vi "PicoScope6000ExampleBlockAdvancedTrigger.vi"() -> ()   [LabVIEW 2010]
uses:
  shared/PicoBuffers.ctl
  shared/Buffer and Transfer Settings.ctl
  shared/Acquisition Settings.ctl
  PicoScope6000Lib/PicoScope6000AnalogChannelSettings.ctl
panel:
  in  "Pulse Width Qualifier Settings":T1={"Direction"=2, "Lower Limit"=0, "Upper Limit"=0, "Pulse Width Type"=4} {"Pulse Width Type" items=["None", "Less Than", "Greater Than", "In Range", "Out of Range"]; "Direction" items=["Rising"=2, "Falling"=3, "Rising Lower"=7, "Falling Lower"=8]}
  in  "Pulse Width Qualifier Conditions":T2 {"Condition Logic" items=["AND", "OR", "XOR"]}
  in  "Trigger Conditions":T3 {"Condition Logic" items=["AND", "OR", "XOR"]}
  in  "Auto Trigger (ms)":i32=1000
  in  "Channel A Trigger Properties":T4={"thresholdUpper"=0, "thresholdUpperHysteresis"=0, "thresholdLower"=0, "thresholdLowerHysteresis"=0, "Threshold Mode"=0, "Direction"=0, "Available"=TRUE} {"Direction" items=["Above / Inside", "Below / Outside", "Rising / Enter", "Falling / Exit", "Rising or Falling / Enter or Exit", "Above Lower", "Below Lower", "Rising Lower", "Falling Lower", "Positive Runt", "Negative Runt"]; "Threshold Mode" items=["Level", "Window"]}
  in  "Write to File":bool
  in  "Channel B Settings":T5={"Enabled"=FALSE, "Coupling"=1, "Range"=6, "Analogue Offset"=0.0, "Bandwidth"=0} {"Bandwidth" items=["Full", "20 MHz"]; "Range" items=["10 mV", "20 mV", "50 mV", "100 mV", "200 mV", "500 mV", "1 V", "2 V", "5 V", "10 V", "20 V", "50 V ", "100 V"]; "Coupling" items=["AC", "DC 1 MOhm", "DC 50 Ohm"]}
  out "Device Info":T6
  out "Properties Panel":T7 {"Max Total Capture Time Available (sec)" format="%.3p"; "Sample Frequency" format="%.3p"; "Sample Internal" format="%.3p"; "Max Samples Available" format="%.3p"; "Total Capture Time (sec)" format="%.3p"}
  in  "Channel A Settings":T5={"Enabled"=TRUE, "Coupling"=1, "Range"=6, "Analogue Offset"=0.0, "Bandwidth"=0} {"Bandwidth" items=["Full", "20 MHz"]; "Range" items=["10 mV", "20 mV", "50 mV", "100 mV", "200 mV", "500 mV", "1 V", "2 V", "5 V", "10 V", "20 V", "50 V ", "100 V"]; "Coupling" items=["AC", "DC 1 MOhm", "DC 50 Ohm"]}
  out "Pico 6000 Units":string
  out "error out":errorcluster
  in  "Data file":path=path "PicoScope6000ExampleBlockAdvanTrig ChA Data"
  in  "Acquisition Settings":T8={"preTriggerSamples"=0, "postTriggerSamples"=5000000, "timebase"=5} {"postTriggerSamples" format="%_6p"; "preTriggerSamples" format="%_6p"}
  in  "Buffer and Transfer Settings":T9={"startIndex"=0, "Samples"=5000000, "Down Sample Ratio"=1, "Down-Sample Mode"=0} {"Down-Sample Mode" items=["RAW none"=2147483648, "None"=0, "Aggregate"=1, "Decimate"=2, "Average"=4]; "Down Sample Ratio" step=1; "Samples" format="%_6p"}
  in  "stop":bool
  out "Analog Channels":cluster{i32, sgl, "Data":dbl[]}[](graph)
  in  "Apply Settings":bool
  out "overflow":i16 format="%04b"
  in  "Serial Number":string
  in  "Use Serial Number":bool
  in  "error in (no error)":errorcluster
  # "Bit 0 = ChA"
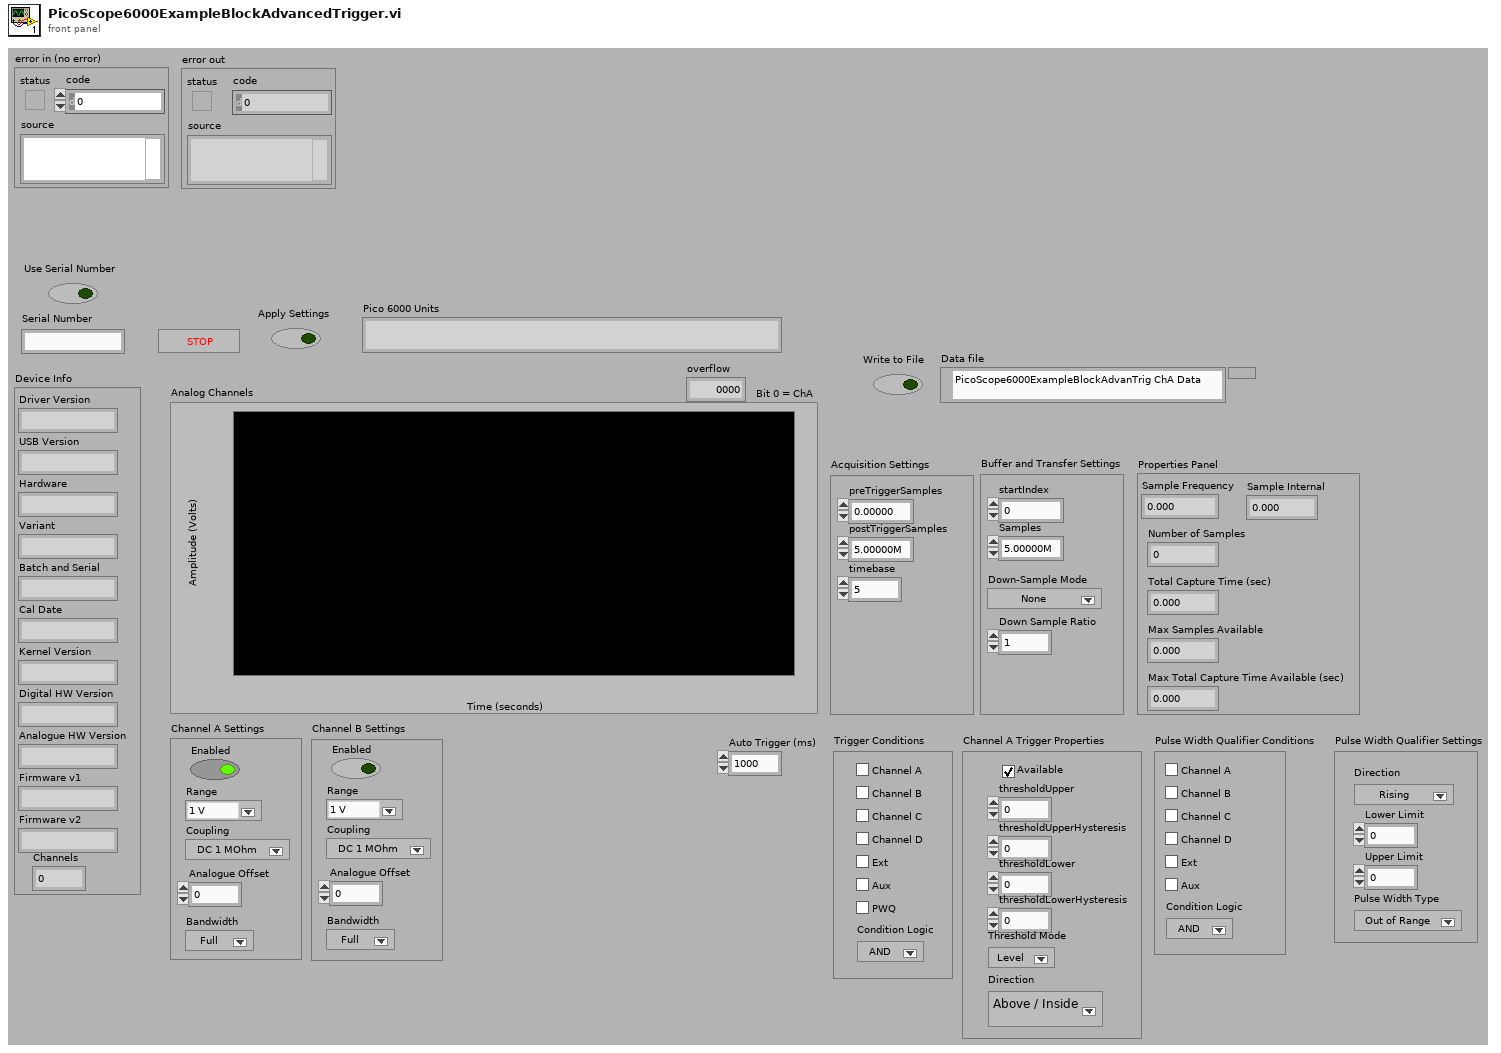
[diagram p1: front panel]
types:
  T1 = cluster{"Direction":i32, "Lower Limit":u32, "Upper Limit":u32, "Pulse Width Type":i32}
  T2 = cluster{"Channel A":bool, "Channel B":bool, "Channel C":bool, "Channel D":bool, "Aux":bool, "Condition Logic":u16, "Ext":bool}
  T3 = cluster{"Channel A":bool, "Channel B":bool, "Channel C":bool, "Channel D":bool, "Aux":bool, "PWQ":bool, "Condition Logic":u16, "Ext":bool}
  T4 = cluster{"thresholdUpper":i16, "thresholdUpperHysteresis":u16, "thresholdLower":i16, "thresholdLowerHysteresis":u16, "Threshold Mode":i32, "Direction":i32, "Available":bool}
  T5 = typedef "PicoScope6000AnalogChannelSettings.ctl" = cluster{"Enabled":bool, "Coupling":u32, "Range":u32, "Analogue Offset":sgl, "Bandwidth":u32}
  T6 = cluster{"Driver Version":string, "USB Version":string, "Hardware":string, "Variant":string, "Batch and Serial":string, "Cal Date":string, "Kernel Version":string, "Digital HW Version":string, "Analogue HW Version":string, "Firmware v1":string, "Firmware v2":string, "Channels":i16}
  T7 = cluster{"Sample Frequency":sgl, "Sample Internal":sgl, "maxSamples":u32, "Number of Samples":u32, "Total Capture Time (sec) ":sgl, "Max Total Capture Time Available (sec)":sgl}
  T8 = typedef "Acquisition Settings.ctl" = cluster{"preTriggerSamples":u64, "postTriggerSamples":u64, "timebase":u32}
  T9 = typedef "Buffer and Transfer Settings.ctl" = cluster{"startIndex":u64, "Samples":u64, "Down Sample Ratio":u64, "Down-Sample Mode":u32}
  T10 = typedef "PicoBuffers.ctl" = cluster{"Max Buffer Pointers":u64[][][], "Min Buffer Pointers":u64[][][], "StreamingDataInfo":cluster{"Channel":u32, "Down-Sample Mode":u32, "PICO_DATA_TYPE":enum32{"PICO_INT8_T", "PICO_INT16_T", "PICO_INT32_T", "PICO_UINT32_T", "PICO_INT64_T", ""}, "Samples":i32, "bufferIndex":u64, "startIndex":i32, "overflow":i16}[][]}
  T11 = enum16{"open", "open or create", "create or replace", "create", "open (read-only)"}
  T12 = cluster{"Channel A Buffer":i16[], "Channel B Buffer":i16[], "Channel C Buffer":i16[], "Channel D Buffer":i16[], "Channel E Buffer":i16[], "Channel F Buffer":i16[], "Channel G Buffer":i16[], "Channel H Buffer":i16[], "Port 0 Buffer":i16[], "Port 1 Buffer":i16[]}[]
  T13 = cluster{"Channel A Buffer":i16[], "Channel B Buffer":i16[], "Channel C Buffer":i16[], "Channel D Buffer":i16[], "Channel E Buffer":i16[], "Channel F Buffer":i16[], "Channel G Buffer":i16[], "Channel H Buffer":i16[], "Port 0 Buffer":i16[], "Port 1 Buffer":i16[]}
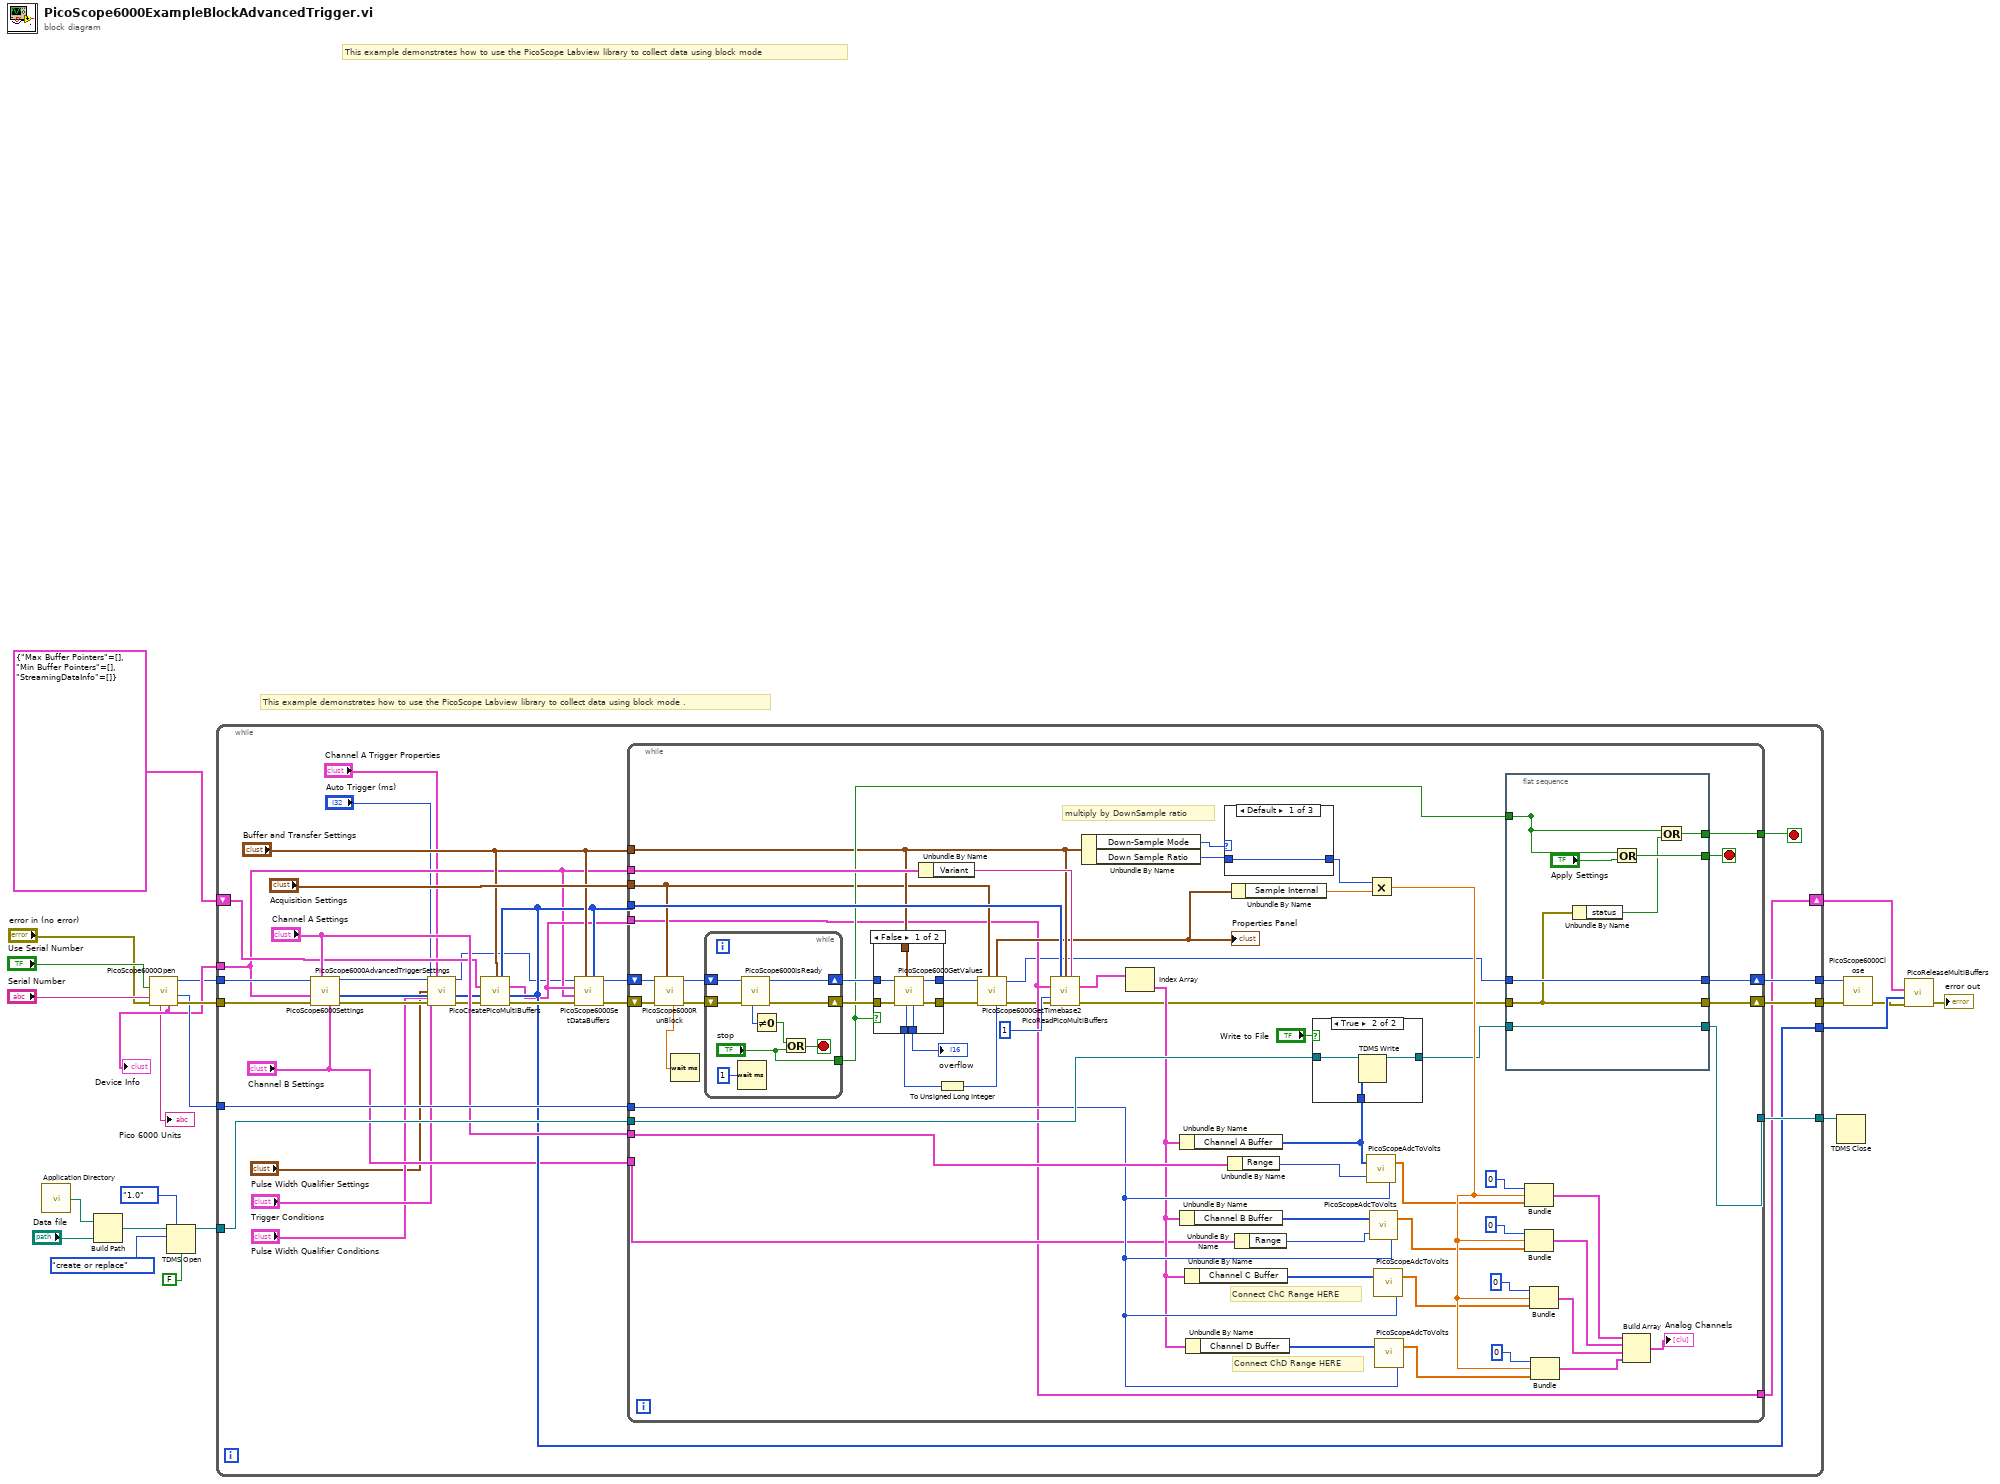
[diagram p0: block diagram]
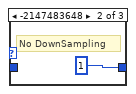
[diagram p4: hidden frame]
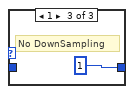
[diagram p5: hidden frame]
diagram:
  # "This example demonstrates how to use the PicoScope Labview library to collect data using block mode ."
  # "This example demonstrates how to use the PicoScope Labview library to collect data using block mode"
  n1 = call <vilib>:"Application Directory.vi"() -> ("Application Directory"=w16:path)
  n2 = Build Path(base path=w16, name or relative path="Data file") -> (appended path=w17:path)
  n3 = call "PicoScope6000Open.vi"("error in (no error)"="error in (no error)", "Serial Number"="Serial Number", "Use Serial Number"="Use Serial Number") -> ("error out"=w9:errorcluster, "Max Adc value"=w7:i16, "handle"=w1:i16, "Device Info"=w6:T6, "Pico 6000 Units"=→"Pico 6000 Units":string)  [unwired: 4 in]
  "Device Info" <- w6
  n4 = TDMS Open(6:FALSE ("disable buffering? (T)"), 7:enum16{"1.0", "2.0"}."1.0" ("file format version (2.0)"), 10:T11."create or replace" ("operation (0:open)"), 11:w17) -> (3:w14:refnum<k34>)  [unwired: 2 in, 1 out]
  n5 = while {
    tunnel: w7 -> [w46]
    tunnel: [w40] -> w23
    tunnel: [w49] -> w15
    tunnel: w14 -> [w52]
    tunnel: w6 -> [w33]
    tunnel: w9 -> [w35]
    tunnel: [w50] -> w3
    tunnel: [w47] -> w12
    shift-right: [w37] -> w22
    shift-left: T10 {"Max Buffer Pointers"=[], "Min Buffer Pointers"=[], "StreamingDataInfo"=[]} ("Data Pointers") -> [w36]
    tunnel: w1 -> [w34]
    stop <- w48 stop-if-true
    n6 = call "PicoScope6000Settings.vi"("Channel B Settings"="Channel B Settings", "Channel A Settings"="Channel A Settings", "error in"=w35, "Device Info"=w33, "handle in"=w34) -> ("error out"=w31:errorcluster, "Enabled array"=w40:i16[], "handle out"=w32:i16)  [unwired: 4 in]
    n7 = call "PicoScope6000AdvancedTriggerSettings.vi"("handle in"=w32, "Channel A Trigger Properties"="Channel A Trigger Properties", "Auto Trigger (ms)"="Auto Trigger (ms)", "Trigger Conditions"="Trigger Conditions", "Pulse Width Qualifier Settings"="Pulse Width Qualifier Settings", "Pulse Width Qualifier Conditions"="Pulse Width Qualifier Conditions", "error in"=w31) -> ("handle out"=w29:i16, "error out"=w30:errorcluster)  [unwired: 7 in]
    n8 = call "PicoCreatePicoMultiBuffers.vi"("Buffer and Transfer Settings"="Buffer and Transfer Settings", "enabled array"=w40, "Data Pointers In"=w36, "error in (no error)"=w30) -> ("Data Pointers"=w39:T10, "error out"=w43:errorcluster)  [unwired: 10 in]
    n9 = call "PicoScope6000SetDataBuffers.vi"("enabled array"=w40, "Buffer and Transfer Settings"="Buffer and Transfer Settings", "error in (no error)"=w43, "Device Info"=w33, "Data Pointers In"=w39, "handle in"=w29) -> ("error out"=w45:errorcluster, "handle out"=w44:i16)  [unwired: 4 in]
    n10 = while {
      tunnel: w39 -> [w58]
      tunnel: "Buffer and Transfer Settings" -> [w69]
      tunnel: w40 -> [w107]
      tunnel: "Channel A Settings" -> [w106]
      tunnel: "Acquisition Settings" -> [w62]
      tunnel: w46 -> [w105]
      tunnel: w33 -> [w102]
      tunnel: [w77] -> w48
      shift-right: [w81] -> w50
      shift-left: w45 -> [w67]
      shift-right: [w75] -> w47
      shift-left: w44 -> [w68]
      tunnel: w52 -> [w113]
      tunnel: [w79] -> w49
      tunnel: "Channel B Settings" -> [w59]
      tunnel: [w58] -> w37
      stop <- w76 stop-if-true
      # "Connect ChD Range HERE"
      # "Connect ChC Range HERE"
      # "multiply by DownSample ratio"
      n11 = call "PicoScope6000RunBlock.vi"("Acquisition Settings"=w62, "error in (no error)"=w67, "handle in"=w68) -> ("error out"=w66:errorcluster, "handle out"=w65:i16, "timeIndisposedMs"=w64:dbl)  [unwired: 5 in, 1 out]
      n12 = Wait (ms)(milliseconds to wait=w64) -> ()  [unwired: 1 out]
      n13 = while {
        shift-right: [w136] -> w73
        shift-left: w66 -> [w140]
        shift-right: [w137] -> w74
        shift-left: w65 -> [w139]
        tunnel: ["stop"] -> w72
        stop <- w142 stop-if-true
        n14 = Wait (ms)(milliseconds to wait=u32 1) -> ()  [unwired: 1 out]
        n15 = call "PicoScope6000IsReady.vi"("error in (no error)"=w140, "handle in"=w139) -> ("error out"=w136:errorcluster, "handle out"=w137:i16, "ready"=w135:i16)  [unwired: 7 in]
        n16 = Not Equal To 0?(x=w135) -> (x != 0?=w143:bool)
        n17 = Or(x=w143, y="stop") -> (x .or. y?=w142:bool)
      }
      n18 = case shown="False" w72 {
        tunnel: w73 -> [w123 w125]
        tunnel: w74 -> [w122 w126]
        tunnel: [w121 w126] -> w55
        tunnel: [w124 w125] -> w56
        tunnel: w69 -> [w120 _]
        tunnel: [w119 _] -> w71
        tunnel: [w118 _] -> w70
        frame False {
          n19 = call "PicoScope6000GetValues.vi"("Buffer and Transfer Settings"=w120, "error in (no error)"=w123, "handle in"=w122) -> ("error out"=w124:errorcluster, "handle out"=w121:i16, "overflow"=w119:i16, "noOfSamples"=w118:u64)  [unwired: 5 in]
        }
        frame True {
        }
      }
      "overflow" <- w71
      n20 = Unbundle By Name(w102) -> ("Variant"=w103:string)
      n21 = To Unsigned Long Integer(number=w70) -> (unsigned 32bit integer=w63:u32)
      n22 = call "PicoScope6000GetTimebase2.vi"("Number of Samples"=w63, "Acquisition Settings"=w62, "error in (no error)"=w56, "handle in"=w55) -> ("error out"=w54:errorcluster, "handle out"=w53:i16, "Properties Panel"=w61:T7)  [unwired: 5 in]
      "Properties Panel" <- w61
      n23 = call "PicoReadPicoMultiBuffers.vi"("enabled array"=w107, "Buffer and Transfer Settings"=w69, "Variant"=w103, "Data Pointers"=w58, "No of Buffers"=1, "error in (no error)"=w54) -> ("MultiBuffers (Max or non-aggregated)"=w112:T12, "error out"=w78:errorcluster)  [unwired: 7 in, 1 out]
      n24 = Unbundle By Name(w69) -> ("Down-Sample Mode"=w110:u32, "Down Sample Ratio"=w111:u64)
      n25 = Index Array(array=w112) -> (element=w82:T13)  [unwired: 1 in]
      n26 = Unbundle By Name(w82) -> ("Channel A Buffer"=w91:i16[])
      n27 = Unbundle By Name(w82) -> ("Channel B Buffer"=w97:i16[])
      n28 = Unbundle By Name(w82) -> ("Channel C Buffer"=w89:i16[])
      n29 = Unbundle By Name(w82) -> ("Channel D Buffer"=w85:i16[])
      n30 = case shown="Default" w110 {
        tunnel: [w144 u64 1 ("Down Sample Ratio") u64 1 ("Down Sample Ratio")] -> w108
        tunnel: w111 -> [w144 _ _]
        frame Default {
        }
        frame -2147483648 {
          # "No DownSampling"
        }
        frame 1 {
          # "No DownSampling"
        }
      }
      n31 = Unbundle By Name(w106) -> ("Range"=w99:u32)
      n32 = Unbundle By Name(w61) -> ("Sample Internal"=w104:sgl)
      n33 = Unbundle By Name(w59) -> ("Range"=w60:u32)
      n34 = case shown="True" "Write to File" {
        tunnel: w113 -> [w114 w117]
        tunnel: w91 -> [_ w116]
        tunnel: [w114 w115] -> w80
        frame False {
        }
        frame True {
          n35 = TDMS Write(0:w117, 9:w116) -> (4:w115:refnum<k34>)  [unwired: 4 in, 3 out]
        }
      }
      n36 = call "PicoScopeAdcToVolts.vi"("Max_adc"=w105, "Range Index"=w99, "Data"=w91) -> ("Data"=w92:dbl[])
      n37 = Multiply(x=w108, y=w104) -> (x*y=w109:sgl)
      n38 = call "PicoScopeAdcToVolts.vi"("Max_adc"=w105, "Range Index"=w60, "Data"=w97) -> ("Data"=w96:dbl[])
      n39 = call "PicoScopeAdcToVolts.vi"("Max_adc"=w105, "Data"=w89) -> ("Data"=w88:dbl[])  [unwired: 1 in]
      n40 = call "PicoScopeAdcToVolts.vi"("Max_adc"=w105, "Data"=w85) -> ("Data"=w84:dbl[])  [unwired: 1 in]
      n41 = flat-sequence {
        tunnel: [w134] -> w76
        tunnel: [w127] -> _
        tunnel: [w131] -> w77
        tunnel: w53 -> [w130]
        tunnel: [w130] -> w75
        tunnel: w78 -> [w129]
        tunnel: [w129] -> w81
        tunnel: [w128] -> w79
        tunnel: w80 -> [w128]
        tunnel: w72 -> [w127]
        frame #0 {
          n42 = Unbundle By Name(w129) -> ("status"=w132:bool)
          n43 = Or(x=w127, y="Apply Settings") -> (x .or. y?=w134:bool)
          n44 = Or(x=w127, y=w132) -> (x .or. y?=w131:bool)
        }
      }
      n45 = Bundle(0, w109, "Data"=w92) -> (w95:cluster{i32, sgl, "Data":dbl[]})  [unwired: 1 in]
      n46 = Bundle(0, w109, "Data"=w96) -> (w94:cluster{i32, sgl, "Data":dbl[]})  [unwired: 1 in]
      n47 = Bundle(0, w109, "Data"=w88) -> (w87:cluster{i32, sgl, "Data":dbl[]})  [unwired: 1 in]
      n48 = Bundle(0, w109, "Data"=w84) -> (w83:cluster{i32, sgl, "Data":dbl[]})  [unwired: 1 in]
      n49 = Build Array(w95, w94, w87, w83) -> (→"Analog Channels":cluster{i32, sgl, "Data":dbl[]}[])
    }
  }
  n50 = TDMS Close(11:w15) -> ()  [unwired: 1 in, 2 out]
  n51 = call "PicoScope6000Close.vi"("error in (no error)"=w3, "handle"=w12) -> ("error out"=w2:errorcluster)  [unwired: 8 in, 1 out]
  n52 = call "PicoReleaseMultiBuffers.vi"("error in (no error)"=w2, "Enabled array"=w23, "Data Pointers"=w22) -> ("error out"=→"error out":errorcluster)  [unwired: 7 in, 1 out]
